vi "USB4704 #1 V1.vi"(6 "TimeOut":i32, 9 "Cycles":i32, 10 "Rate":i32, 11 "Start/Stop":bool) -> (0 "error out":errorcluster, 3 "data out(DDT)":dynamicdata(waveform))   [LabVIEW 2013]
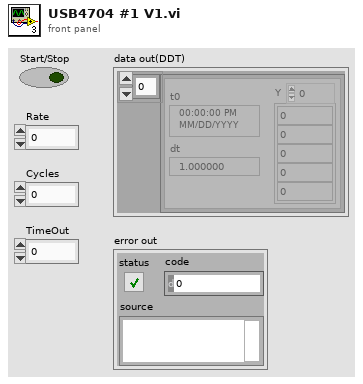
[diagram p1: front panel]
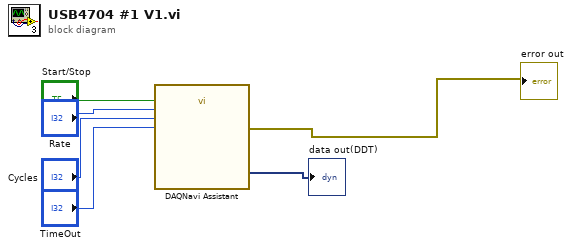
[diagram p0: block diagram]
diagram:
  n1 = call "DAQNavi Assistant"("stop(true)"="Start/Stop", "conversion rate(Hz)"="Rate", "samples"="Cycles", "time out(10s)"="TimeOut") -> ("error out"=→"error out":errorcluster, "data out(DDT)"=→"data out(DDT)":dynamicdata)  [unwired: 22 in]
